vi "addSubsystem.vi"(8 "error in (no error)":errorcluster, 10 "Subsystem To Add":refnum<class "Subsystem.lvclass">, 11 "Subsystem in":refnum<class "Subsystem.lvclass">) -> (0 "error out":errorcluster, 3 "Subsystem out":refnum<class "Subsystem.lvclass">)   [LabVIEW 2017, in "Subsystem.lvclass"]
uses:
  <userlib>/836-Library/Robot/Subsystem/Subsystem.lvclass
  <userlib>/836-Library/Robot/Subsystem/Subsystem.lvclass/Subsystem.ctl
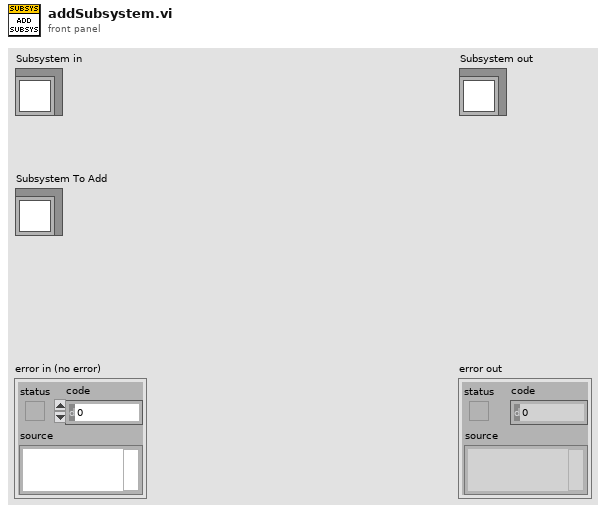
[diagram p1: front panel]
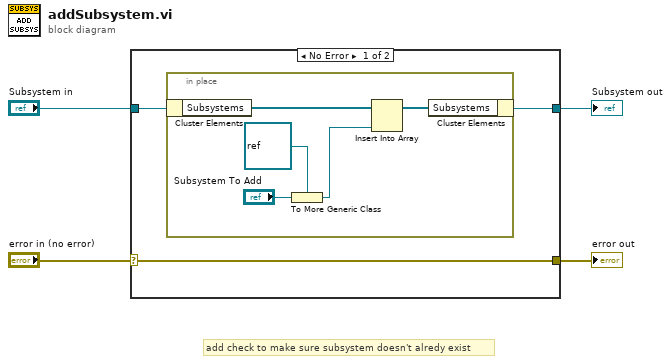
[diagram p0: block diagram]
diagram:
  # "add check to make sure subsystem doesn't alredy exist"
  n1 = case shown="No Error" "error in (no error)" {
    selector: "error in (no error)" -> [w7 w14]
    tunnel: [w7 w14] -> w3
    tunnel: [w5 w13] -> w1
    tunnel: "Subsystem in" -> [w6 w13]
    frame No Error {
      n2 = in-place {
        n3 = in-place-cluster #1(w6) -> ("Subsystems"=w12:refnum<class>[])
        n4 = To More Generic Class(target class=refnum<class> refnum ("LabVIEW Object"), reference="Subsystem To Add") -> (generic class reference=w8:refnum<class>)
        n5 = Insert Into Array(array=w12, new element=w8) -> (w11:refnum<class>[])  [unwired: 1 in]
        n6 = in-place-cluster #1("Subsystems"=w11) -> (w5:refnum<class "Subsystem.lvclass">)
      }
    }
    frame Error {
    }
  }
  "error out" <- w3
  "Subsystem out" <- w1
